vi "Raise D arm.vi"(8 "Power":i8=10, 10 "Rotation":i32=100, 11 "EV3 in":T1) -> (3 "EV3 out":T1)   [LabVIEW 2016]
uses:
  <vilib>/NXT/Subs/LVHSConnector.ctl
  <vilib>/NXT/LegoClasses/BrickReference/BrickReference.lvclass
  <vilib>/NXT/Block Support/NXT_OutputPort.ctl
  <vilib>/NXT/NXTIO Xnodes/NXTIONodeSubVIs/LEGOResetMotors.vi
  <vilib>/NXT/NXTIO Xnodes/NXTIONodeSubVIs/NXTMotorRunDistance.vi
  <vilib>/NXT/NXTIO Xnodes/AddressXNode/NXTIOAddress.xnode
  <vilib>/NXT/NXTIO Xnodes/NXTIOXNode/NXTIO.xnode
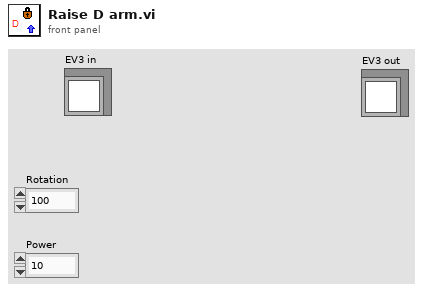
[diagram p1: front panel]
types:
  T1 = typedef "LVHSConnector.ctl" = refnum<class "BrickReference.lvclass">
  T2 = typedef "NXT_OutputPort.ctl" = u8
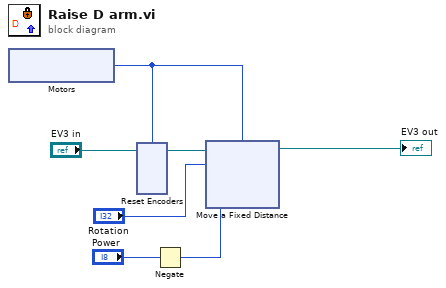
[diagram p0: block diagram]
diagram:
  n1 = xnode "Motors"() -> ("Motor"=w7:T2)
  n2 = xnode "Reset Encoders"("Motors"=w7, "NXT/EV3"="EV3 in") -> ("NXT/EV3"=w4:T1)
  n3 = Negate(x="Power") -> (-x=w1:i8)
  n4 = xnode "Move a Fixed Distance"("Speed 1"=w1, "Distance 1"="Rotation", "Motors"=w7, "NXT/EV3"=w4) -> ("NXT/EV3"=→"EV3 out":T1)
